vi "FindSingleCircleEdge (SubVI).vi"(5 "Circle Finding Options":T7={"Search  Direction"=1, "Edge Options"={"Edge Polarity"=2, "Kernel Size"=3, "Width"=3, "Minimum Edge Strength"=10.0, "Interpolation Type"=enum."Bilinear Fixed", "Data Processing Method"=enum."Average"}, "Show Search Area"=FALSE, "Show Search Lines"=FALSE, "Show Edges Found"=FALSE, "Show Result"=TRUE, "Search Area Color"=65280, "Search Lines Color"=255, "Edge Locations Color"=16776960, "Result Color"=65511, "Overlay Group Name"=""} {"Search  Direction" items=["Outside to Inside", "Inside to Outside"]; "Edge Options"."Edge Polarity" items=["All Edges", "Rising Edges", "Falling Edges"]; "Edge Options"."Minimum Edge Strength" format="%.2f"; "Edge Options"."Width" step=2; "Edge Options"."Kernel Size" step=2}, 6 "Circle Fit Options":T4={"Process"=enum."Get Best Edge", "Step Size"=3.0, "Max Pixel Radius"=3}, 7 "Circle ROI Descriptor":T3={"Global Rectangle"=[675, 567, 1751, 1642], "Contours"=[{"ID"=enum."External", "Type"=7, "Coordinates"=[1212, 1104, 85, 537, 0, 0]}]} {"Contours"."Type" items=["No Selection", "Point", "Line", "Rectangle", "Oval", "Polygon", "Freehand Region", "Annulus", "Unused2", "Unused3", "Broken Line", "Freehand Line", "Rotated Rectangle"]}, 8 "error in (no error)":errorcluster, 9 "Search Image in":T1, 10 "Pattern Match Settings":T8={"Algorithm"=2, "Number of Matches Requested"=1, "Minimum Match Score"=800.0, "SubPixel Accuracy"=TRUE, "Rotation Angle Ranges"=[], "Show Search Area"=FALSE, "Show Result"=TRUE} {"Rotation Angle Ranges"."End" format="%.1f"; "Rotation Angle Ranges"."Start" format="%.1f"; "Minimum Match Score" min=0 max=1000 format="%.2f"; "Number of Matches Requested" min=1; "Algorithm" items=["All", "Low Discrepancy Sampling", "Grayscale Value Pyramid", "Gradients Pyramid"]}, 11 "Template in":T1) -> (0 "error out":errorcluster, 2 "Fitted Circle":T2, 3 "Search image out":T1)   [LabVIEW 2016]
uses:
  <vilib>/vision/Measure.llb/Edge Options.ctl
  <vilib>/vision/Measure.llb/Edge Polarity.ctl
  <vilib>/vision/Image Controls.llb/IMAQ Image.ctl
  <vilib>/vision/NI_Vision_Development_Module.lvlib
panel:
  # "(3) Find and fit the circle"
  # "(4) Export the results"
  # "(1) Perform a pattern match to a template circle"
  # "(2) Create a dynamic Region of Interest (ROI) based on the coordinates\nof the pattern match result"
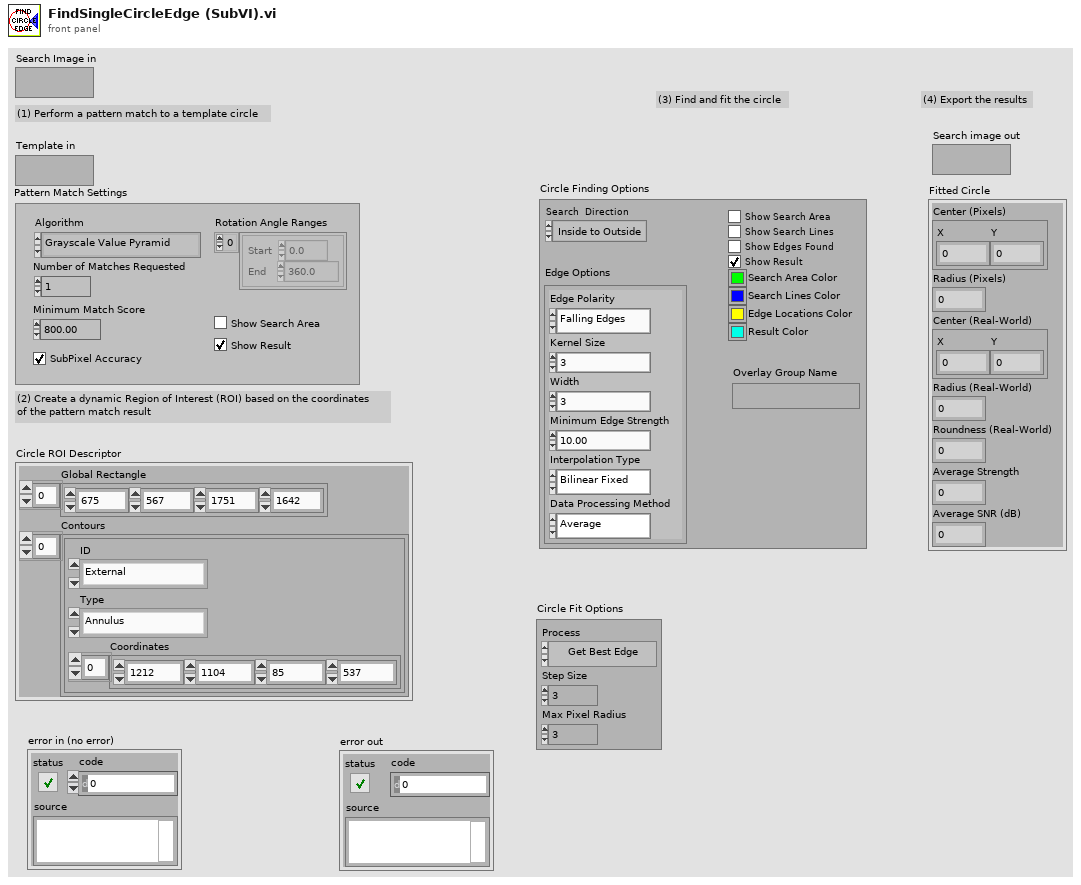
[diagram p1: front panel]
types:
  T1 = typedef "IMAQ Image.ctl" = refnum<image>
  T2 = cluster{"Center (Pixels)":cluster{"X":sgl, "Y":sgl}, "Radius (Pixels)":dbl, "Center (Real-World)":cluster{"X":sgl, "Y":sgl}, "Radius (Real-World)":dbl, "Roundness (Real-World)":dbl, "Average Strength":dbl, "Average SNR (dB)":dbl}
  T3 = cluster{"Global Rectangle":i32[], "Contours":cluster{"ID":enum32{"External", "Internal"}, "Type":u32, "Coordinates":i32[]}[]}
  T4 = cluster{"Process":enum16{"Get First Edge", "Get First + Last Edge", "Get All Edges", "Get Best Edge"}, "Step Size":dbl, "Max Pixel Radius":i32}
  T5 = typedef "Edge Options.ctl" = cluster{"Edge Polarity":T6, "Kernel Size":u32, "Width":u32, "Minimum Edge Strength":sgl, "Interpolation Type":enum32{"Zero Order", "Bilinear", "Quadratic", "Cubic", "Bilinear Fixed"}, "Data Processing Method":enum32{"Average", "Median"}}
  T6 = typedef "Edge Polarity.ctl" = u32
  T7 = cluster{"Search  Direction":u32, "Edge Options":T5, "Show Search Area":bool, "Show Search Lines":bool, "Show Edges Found":bool, "Show Result":bool, "Search Area Color":u32, "Search Lines Color":u32, "Edge Locations Color":u32, "Result Color":u32, "Overlay Group Name":string}
  T8 = cluster{"Algorithm":i32, "Number of Matches Requested":i32, "Minimum Match Score":sgl, "SubPixel Accuracy":bool, "Rotation Angle Ranges":cluster{"Start":sgl, "End":sgl}[], "Show Search Area":bool, "Show Result":bool}
  T9 = cluster{"Position":cluster{"x":sgl, "y":sgl}, "Angle":sgl, "Scale":sgl, "Score":sgl, "Bounding Box":cluster{"x":sgl, "y":sgl}[]}[]
  T10 = cluster{"Global Rectangle":i32[], cluster{"ID":enum32{"External", "Internal"}, "Type":u32, "Coordinates":i32[]}[]}
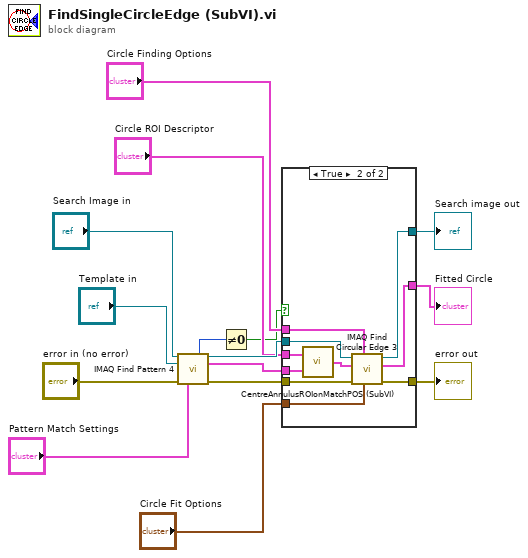
[diagram p0: block diagram]
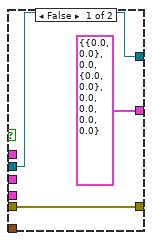
[diagram p2: hidden frame]
diagram:
  n1 = call "IMAQ Find Pattern 4"("Image"="Search Image in", "Template"="Template in", "error in"="error in (no error)", "Settings"="Pattern Match Settings") -> ("Number of Matches"=w2:i32, "Image Out"=w11:T1, "Matches (pixel)"=w10:T9, "error out"=w12:errorcluster)  [unwired: 5 in, 3 out]
  n2 = Not Equal To 0?(x=w2) -> (x != 0?=w1:bool)
  n3 = case shown="True" w1 {
    tunnel: [T2 {"Center (Pixels)"={"X"=0.0, "Y"=0.0}, "Radius (Pixels)"=0.0, "Center (Real-World)"={"X"=0.0, "Y"=0.0}, "Radius (Real-World)"=0.0, "Roundness (Real-World)"=0.0, "Average Strength"=0.0, "Average SNR (dB)"=0.0} ("Fitted Circle") w28] -> w15
    tunnel: [w18 w27] -> w14
    tunnel: [w17 w26] -> w13
    tunnel: w12 -> [w17 w25]
    tunnel: w11 -> [w18 w24]
    tunnel: w10 -> [_ w22]
    tunnel: "Circle ROI Descriptor" -> [_ w21]
    tunnel: "Circle Fit Options" -> [_ w20]
    tunnel: "Circle Finding Options" -> [_ w19]
    frame False {
    }
    frame True {
      n4 = call "CentreAnnulusROIonMatchPOS (SubVI).vi"("Matches (pixel)"=w22, "Annulus ROI Descriptor"=w21) -> ("Annulus ROI Descriptor centred on match position"=w23:T10)
      n5 = call "IMAQ Find Circular Edge 3"("Circle Fit Options"=w20, "Options"=w19, "error in (no error)"=w25, "ROI Descriptor"=w23, "Image"=w24) -> ("error out"=w26:errorcluster, "Fitted Circle"=w28:T2, "Image Out"=w27:T1)  [unwired: 2 in, 2 out]
    }
  }
  "Fitted Circle" <- w15
  "Search image out" <- w14
  "error out" <- w13
